vi "Main Editor UI.vi"() -> ()   [LabVIEW 2015, in "SystemLink editor node.lvclass"]
doc: "This is the main view for configuration the behavior of a module in the DCAF standard editor."
uses:
  SystemLink editor node.lvclass
  <vilib>/NI/Configuration Framework/Node/NodeRef.ctl
  <vilib>/NI/Configuration Framework/Node/NISE_CEF_Node.lvclass
  <vilib>/NI/AMC/Message Queue.ctl
  <vilib>/NI/AMC/Message.ctl
  <vilib>/NI/Tools/Keyed Array/KeyedArray.ctl
  <vilib>/NI/Configuration Framework/Node/UserEventRef.ctl
  <vilib>/NI/Configuration Framework/Controls/EventCluster.ctl
  <vilib>/NI/DCAF UI Toolkit/Controls/Configure.ctl
  <vilib>/NI/DCAF UI Toolkit/Controls/Add.ctl
  <vilib>/NI/DCAF UI Toolkit/Controls/Remove.ctl
  <vilib>/NI/Configuration Framework/Node/StopEvent.ctl
  <vilib>/NI/Configuration Framework/Node/RefreshUIEvent.ctl
  <vilib>/NI/Configuration Framework/Node/CacheState.ctl
  <vilib>/NI/Configuration Framework/Node/NodeChangeEvent.ctl
  module/configuration/Permissions Enum.ctl
  <vilib>/NI/DCAF/Tag Editor Core/Table API/Available Tag Menu/channel action event.ctl
  <vilib>/NI/DCAF/Tag Editor Core/Table API/Available Tag Menu/dialog output action.ctl
  <vilib>/NI/Tag Bus Module Framework/channel/TBM channel.lvclass
  <vilib>/NI/Tag Bus/tag/tag descriptor.lvclass
  <vilib>/NI/DCAF/Tag Editor Core/Table API/Table Manager/Call Back Ref Type Def.ctl
  <vilib>/NI/DCAF/Tag Editor Core/Configuration Editor/Classes/Engine Parent/Engine Parent Editor Node.lvclass
  <vilib>/NI/DCAF/Tag Editor Core/Configuration Editor/Classes/Module editor node/module editor node.lvclass
  <vilib>/NI/DCAF UI Toolkit/Controls/Import.ctl
  <vilib>/NI/DCAF UI Toolkit/Controls/Export.ctl
  module/configuration/Data Tag Type.ctl
  <vilib>/NI/DCAF/Tag Editor Core/Table API/Table Manager/references.ctl
  module/configuration/SystemLink configuration.lvclass
  module/configuration/SystemLink configuration.lvclass/SystemLink configuration.ctl
  <vilib>/Utility/miscctls.llb/LVPositionTypeDef.ctl
  module/configuration/Read Connection Configuration.vi
  <vilib>/NI/Configuration Framework/serializable configuration/NISE_CEF_serializable configuration.lvclass
  <vilib>/NI/DCAF/Tag Editor Core/Table API/Listbox/Multi Column Listbox.lvclass
  <vilib>/NI/Configuration Framework/NISE_CEF_TreeControl.lvlib
  <vilib>/NI/Tools/Keyed Array/Tools_KeyedArray.lvlib
  <vilib>/NI/AMC/AMC.lvlib
  <vilib>/NI/DCAF/Tag Editor Core/Table API/Table Manager.lvlib
  <vilib>/NI/DCAF/Tag Editor Core/Table API/Table Manager/Table Manager.lvclass
  <vilib>/NI/DCAF UI Toolkit/Controls/DCAF UI Elements.lvlib
panel:
  in  "Data Type":T1
  in  "user event out":refnum<user-event>
  in  "Permissions":T2
  in  "node change":T3
  in  "cache state":T4
  in  "refresh UI":T5
  in  "stop event":T6
  in  "Tab Control":T7(tab)=enum."Connection Configuration"
  in  "Remove Button":T8
  in  "Add Button":T9
  in  "Table":i32(listbox)
  in  "settings":T10
  in  "Configuration":T11={"Configuration ID"="", "HTTP"={"Verify Server?"=TRUE, "Server URL"="", "CA Certificate File"="", "User Info"={"Username"="", "Password"=""}, "API Key"=""}}
  in  "Connection Type":T12(ring)
  in  "Export":T13
  in  "Import":T14
  in  "user event":T15
  in  "main queue":T16
  in  "node ref":T17
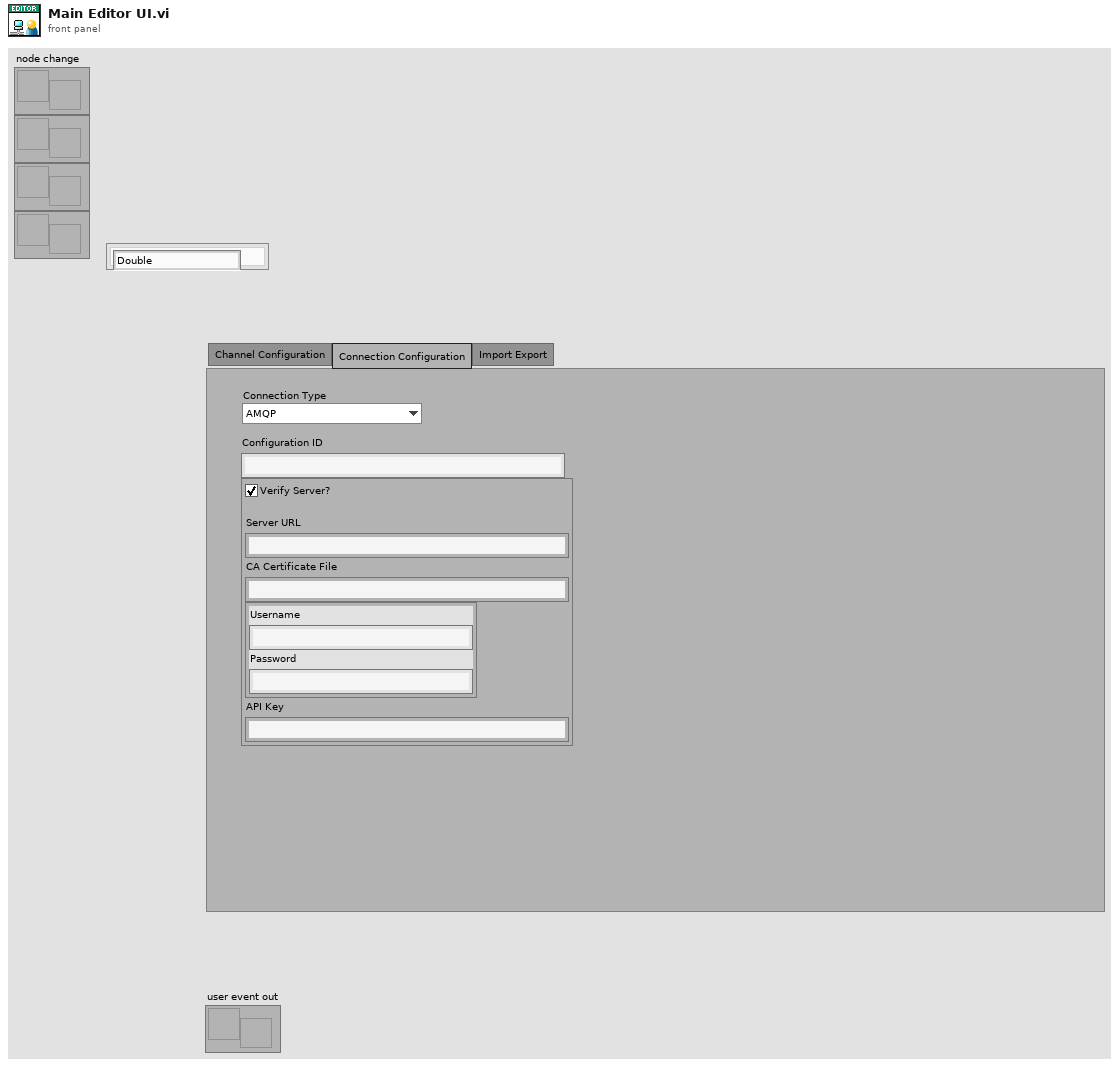
[diagram p1: front panel]
types:
  T1 = typedef "SystemLink configuration.lvclass/Data Tag Type.ctl" = enum16{"Double", "Single", "I32", "I16", "I8", "U64", "U32", "U16", "U8", "Boolean", "String", "Timestamp"}
  T2 = typedef "SystemLink configuration.lvclass/Permissions Enum.ctl" = enum16{"Read from SystemLink", "Write to SystemLink"}
  T3 = typedef "NISE_CEF_Node.lvclass/NodeChangeEvent.ctl" = refnum<user-event>
  T4 = typedef "NISE_CEF_Node.lvclass/CacheState.ctl" = refnum<user-event>
  T5 = typedef "NISE_CEF_Node.lvclass/RefreshUIEvent.ctl" = refnum<user-event>
  T6 = typedef "NISE_CEF_Node.lvclass/StopEvent.ctl" = refnum<user-event>
  T7 = enum32{"Channel Configuration", "Connection Configuration", "Import Export"}
  T8 = typedef "DCAF UI Elements.lvlib/Remove.ctl" = bool
  T9 = typedef "DCAF UI Elements.lvlib/Add.ctl" = bool
  T10 = typedef "DCAF UI Elements.lvlib/Configure.ctl" = bool
  T11 = cluster{"Configuration ID":string, "HTTP":cluster{"Verify Server?":bool, "Server URL":string, "CA Certificate File":string, "User Info":cluster{"Username":string, "Password":string}, "API Key":string}}
  T12 = enum16{"AMQP", "HTTP", "API Key (SystemLink Cloud)"}
  T13 = typedef "DCAF UI Elements.lvlib/Export.ctl" = bool
  T14 = typedef "DCAF UI Elements.lvlib/Import.ctl" = bool
  T15 = typedef "NISE_CEF_Node.lvclass/UserEventRef.ctl" = refnum<user-event>
  T16 = typedef "AMC.lvlib/Message Queue.ctl" = refnum<queue>
  T17 = typedef "NISE_CEF_Node.lvclass/NodeRef.ctl" = refnum<data-value>
  T18 = typedef "Table Manager.lvlib/Table Manager.lvclass/references.ctl" = cluster{"stop event":T6, "refresh UI":T5, "cache state":T4, "node change":T3, "user event out":refnum<user-event>, "main queue":T16, "user event":T15}
  T19 = typedef "LVPositionTypeDef.ctl" = cluster{"Left":i32, "Top":i32}
  T20 = typedef "Table Manager.lvlib/Table Manager.lvclass/object ref.ctl" = cluster{"engine":refnum<data-value>, "Node Ref":refnum<data-value>}
  T21 = typedef "Table Manager.lvlib/Column.lvclass/Column Descriptor.ctl" = cluster{"name":string, "caption":string, "Column Type":T22, "Params":string, "AutoSizeMode":i32, "FillWeight":sgl, "MinWidth":u32, "tooltip":string, "Enum Reference":refnum<vi>, "Channel suffix":string, "Read Only":bool, "Call Back VI":T23, "DT Dependency":i32, "name dependency":i32, "data type":T24, "Custom Column":refnum<class "Column.lvclass">}
  T22 = typedef "Table Manager.lvlib/Column.lvclass/Column Type.ctl" = enum16{"String", "Mapping", "Enum", "Custom"}
  T23 = typedef "Table Manager.lvlib/Table Manager.lvclass/Call Back Ref Type Def.ctl" = refnum<vi>
  T24 = typedef "tag bus.lvlib/tag descriptor.lvclass/Data Type.ctl" = enum16{"Double", "Single", "I64", "I32", "I16", "I8", "U64", "U32", "U16", "U8", "Boolean", "String", "Array of Double", "Array of Single", "Array of I64", "Array of I32", "Array of I16", "Array of I8", "Array of U64", "Array of U32", "Array of U16", "Array of U8", "Array of Boolean", "Array of String"}
  T25 = typedef "SystemLink configuration.lvclass/Connection Configuration.ctl" = cluster{"Connection Type":T26, "AMQP":cluster{"Configuration ID":string}, "HTTP":cluster{"Verify Server?":bool, "Server URL":string, "CA Certificate File":string, "User Info":cluster{"Username":string, "Password":string}, "API Key":string}}
  T26 = typedef "SystemLink configuration.lvclass/Connection Type.ctl" = enum16{"AMQP", "HTTP", "API Key (SystemLink Cloud)"}
  T27 = cluster{"Verify Server?":bool, "Server URL":string, "CA Certificate File":string, "User Info":cluster{"Username":string, "Password":string}, "API Key":string}
  T28 = typedef "Table Manager.lvlib/Table Manager.lvclass/Table Events.ctl" = cluster{"Menu Selection":refnum<user-event>}
  T29 = enum8{"Enabled", "Disabled", "Disabled and Grayed Out"}
  T30 = cluster{"AMQP Specific":refnum<vi>, "HTTP Generic":refnum<vi>, "HTTP Specific":refnum<vi>, "API Key Specific":refnum<vi>}
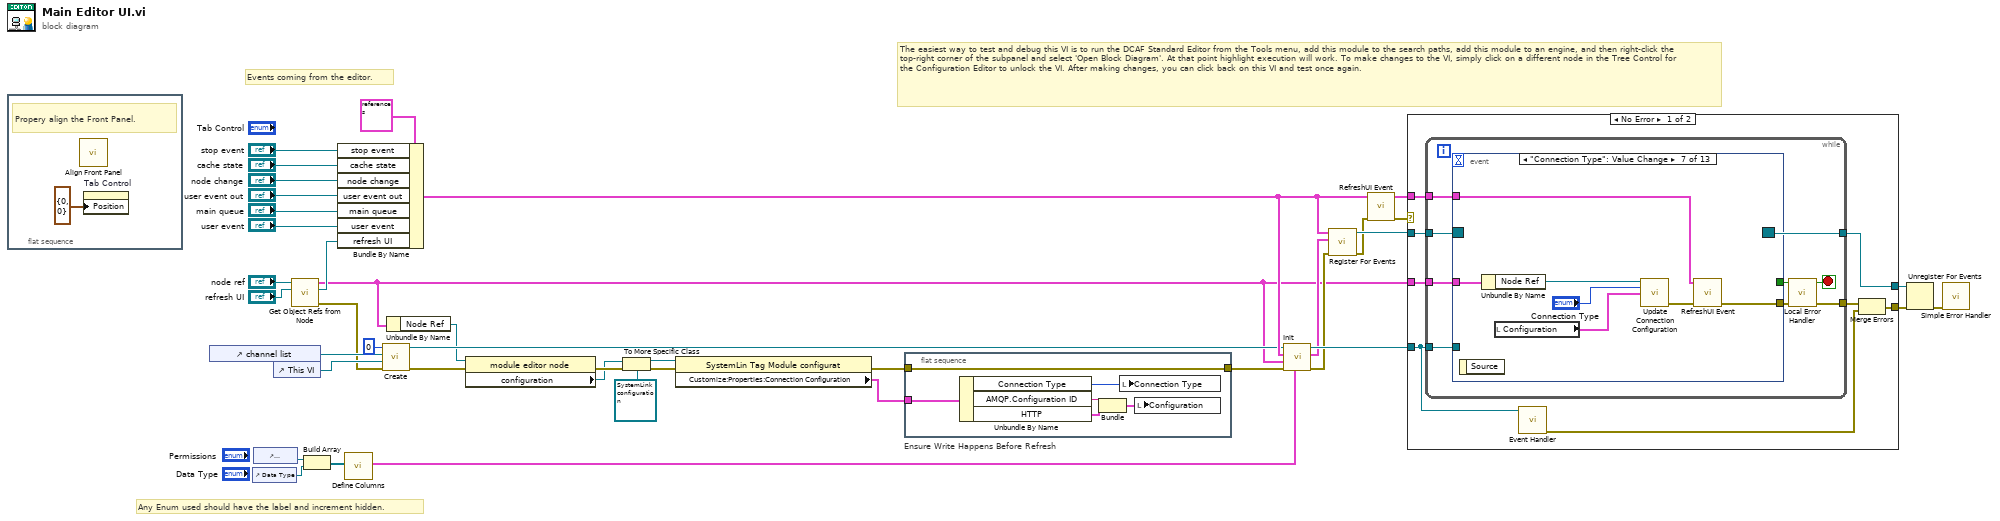
[diagram p0: block diagram]
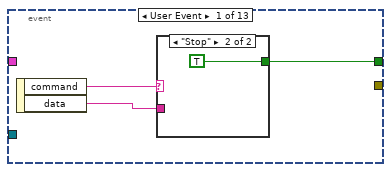
[diagram p2: hidden frame]
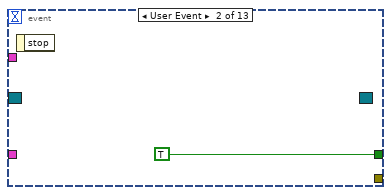
[diagram p4: hidden frame]
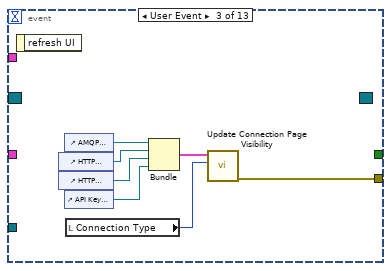
[diagram p5: hidden frame]
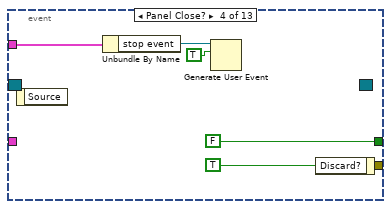
[diagram p6: hidden frame]
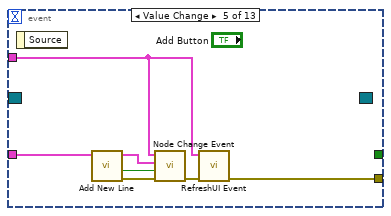
[diagram p7: hidden frame]
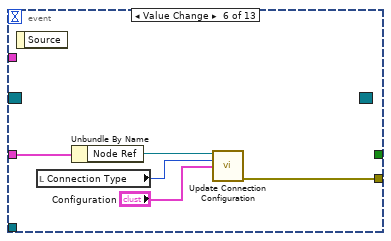
[diagram p8: hidden frame]
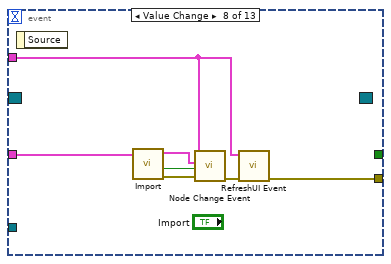
[diagram p9: hidden frame]
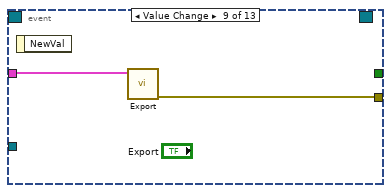
[diagram p10: hidden frame]
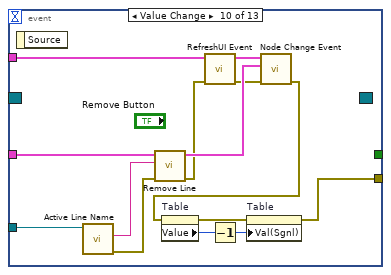
[diagram p11: hidden frame]
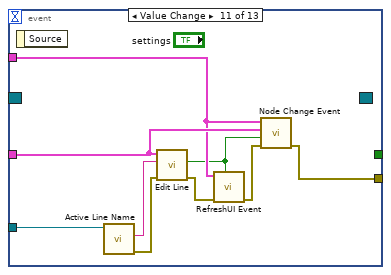
[diagram p12: hidden frame]
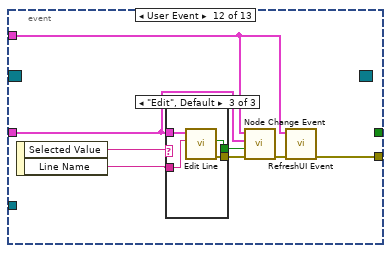
[diagram p13: hidden frame]
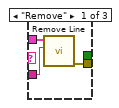
[diagram p14: hidden frame]
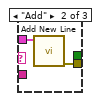
[diagram p15: hidden frame]
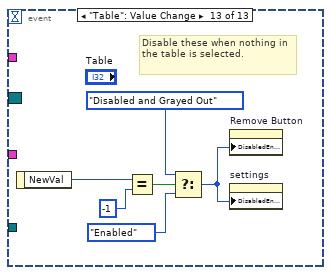
[diagram p16: hidden frame]
diagram:
  # "The easiest way to test and debug this VI is to run the DCAF Standard Editor from the Tools menu, add this module to the search paths, add this module to an engine, and then right-click the top-right corner of the subpanel and select 'Open Block Diagram'. At that point highlight execution will work. To make changes to the VI, simply click on a different node in the Tree Control for the Configuration Editor to unlock the VI. After making changes, you can click back on this VI and test once again."
  # "Any Enum used should have the label and increment hidden."
  # "Events coming from the editor."
  n1 = flat-sequence {
    frame #0 {
      # "Propery align the Front Panel."
      n2 = call <vilib>:"Align Front Panel.vi"() -> ()  [unwired: 10 in, 2 out]
      n3 = property on="Tab Control" class="TabCtl (strict)"("Position"=T19 {"Left"=0, "Top"=0}) -> ()  [unwired: 2 in, 2 out]
    }
  }
  n4 = control-ref of="channel list"() -> (w19:refnum<vi>)
  n5 = control-ref of="Data Type"() -> (w11:refnum<vi>)
  n6 = control-ref of="Permissions"() -> (w27:refnum<vi>)
  n7 = control-ref of="This VI"() -> (w17:refnum<vi>)
  n8 = call "Get Object Refs from Node.vi"("Refresh UI"="refresh UI", "Data Value Reference in"="node ref") -> ("error out"=w14:errorcluster, "Refresh UI out"=w12:T5, "References"=w9:T20)  [unwired: 7 in]
  n9 = Build Array(w27, w11) -> (w26:refnum<vi>[])
  n10 = Bundle By Name(cluster=T18 {"stop event"=refnum, "refresh UI"=refnum, "cache state"=refnum, "node change"=refnum, "user event out"=refnum, "main queue"=refnum, "user event"=refnum} ("References"), "stop event"="stop event", "cache state"="cache state", "node change"="node change", "user event out"="user event out", "main queue"="main queue", "user event"="user event", "refresh UI"=w12) -> (w28:T18)
  n11 = call "Define Columns.vi"("Enum Array"=w26) -> ("Column Definition"=w30:T21[])  [unwired: 10 in]
  n12 = call <vilib>:"Create.vi"("error in (no error)"=w14, "Top VI"=w17, "Listbox"=w19, "Index"=0) -> ("error out"=w15:errorcluster, "reference out"=w16:refnum<class "Multi Column Listbox.lvclass">)  [unwired: 6 in]
  n13 = Unbundle By Name(w9) -> ("Node Ref"=w8:refnum<data-value>)
  n14 = property class="module editor node"(reference=w8, error in=w15) -> (error out=w10:errorcluster, "configuration"=w6:refnum<class "NISE_CEF_serializable configuration.lvclass">)  [unwired: 1 out]
  n15 = To More Specific Class(target class=refnum<class "SystemLink configuration.lvclass"> refnum ("SystemLin Tag Module configuration"), reference=w6, error in=w10) -> (specific class reference=w4:refnum<class "SystemLink configuration.lvclass">, error out=w7:errorcluster)
  n16 = property class="SystemLin Tag Module configurat"(reference=w4, error in=w7) -> (error out=w2:errorcluster, "Customize:Properties:Connection Configuration"=w3:T25)  [unwired: 1 out]
  n17 = flat-sequence "Ensure Write Happens Before Refresh" {
    tunnel: w3 -> [w48]
    tunnel: w2 -> [w46]
    tunnel: [w46] -> w1
    frame #0 {
      n18 = Unbundle By Name(w48) -> ("Connection Type"=w47:T26, "AMQP.Configuration ID"=w44:string, "HTTP"=w43:T27)
      n19 = Bundle("Configuration ID"=w44, "HTTP"=w43) -> (w45:T11)  [unwired: 1 in]
      n20 = local write "Connection Type"(w47) -> ()
      n21 = local write "Configuration"(w45) -> ()
    }
  }
  n22 = call-dynamic "Init.vi"("Column Descriptors"=w30, "error in (no error)"=w1, "Node object refs"=w9, "Event References"=w28, "Multi Column Listbox in"=w16) -> ("error out"=w21:errorcluster, "Table Events"=w20:T28, "Multi Column Listbox out"=w25:refnum<class "Multi Column Listbox.lvclass">)  [unwired: 4 in]
  n23 = call "Register For Events.vi"("error in"=w21, "Table Events"=w20, "References"=w28) -> ("error out"=w23:errorcluster, "Event Registration Refnum"=w31:refnum<event-registration>)  [unwired: 7 in]
  n24 = call "RefreshUI Event.vi"("error in (no error)"=w23, "References in"=w28) -> ("error out"=w22:errorcluster, "References out"=w29:T18)  [unwired: 8 in]
  n25 = case shown="No Error" w22 {
    selector: w22 -> [_ w156]
    tunnel: w31 -> [w56 w155]
    tunnel: [w55 w155] -> w41
    tunnel: [w49 w156] -> w40
    tunnel: w29 -> [w54 _]
    tunnel: w9 -> [w53 _]
    tunnel: w25 -> [w52 _]
    frame No Error {
      n26 = while {
        tunnel: w56 -> [w65]
        tunnel: [w64] -> w55
        tunnel: [w61] -> w50
        tunnel: w54 -> [w59]
        tunnel: w53 -> [w58]
        tunnel: w52 -> [w57]
        stop <- w63 stop-if-true
        n27 = event shown="[6] \"Connection Type\": Value Change" {
          selector: w65 -> [_ _ _ _ _ _ _ _ _ _ _ _ _]
          dyn-events: [_ _ _ _ _ _ _ _ _ _ _ _ _] -> w64
          timeout: _ -> [_ _ _ _ _ _ _ _ _ _ _ _ _]
          tunnel: [w68 TRUE _ FALSE _ _ _ _ _ _ _ _ _] -> w62
          tunnel: [_ _ w71 _ w83 w91 w96 w106 w109 w111 w131 w137 _] -> w60
          tunnel: w59 -> [_ _ _ w79 w87 _ w95 w103 _ w122 w126 w133 _]
          tunnel: w58 -> [_ _ _ _ w88 w93 w99 w105 w108 w121 w129 w134 _]
          tunnel: w57 -> [_ _ _ _ _ _ _ _ _ w117 w130 _ _]
          event User Event {
            n28 = event-data() -> ("command"=w67:string, "data"=w66:string)  [unwired: 1 in]
            n29 = case shown="\"Stop\"" w67 {
              tunnel: [_ TRUE] -> w68
              tunnel: w66 -> [_ _]
              frame Default {
              }
              frame "Stop" {
              }
            }
          }
          event User Event {
            n30 = event-data() -> ()  [unwired: 1 in, 1 out]
          }
          event User Event {
            n31 = event-data() -> ()  [unwired: 1 in, 1 out]
            n32 = control-ref of="HTTP Generic"() -> (w76:refnum<vi>)
            n33 = control-ref of="HTTP Specific"() -> (w75:refnum<vi>)
            n34 = control-ref of="AMQP Specific"() -> (w77:refnum<vi>)
            n35 = control-ref of="API Key Specific"() -> (w74:refnum<vi>)
            n36 = local read "Connection Type"() -> (w72:T12)
            n37 = Bundle("AMQP Specific"=w77, "HTTP Generic"=w76, "HTTP Specific"=w75, "API Key Specific"=w74) -> (w73:T30)  [unwired: 1 in]
            n38 = call "Update Connection Page Visibility.vi"("Connection Type"=w72, "Config References"=w73) -> ("error out"=w71:errorcluster)  [unwired: 9 in]
          }
          event Panel Close? {
            n39 = event-data() -> ()  [unwired: 1 in, 1 out]
            n40 = Unbundle By Name(w79) -> ("stop event"=w78:T6)
            n41 = Generate User Event(user event=w78, event data cluster=TRUE ("event data")) -> ()  [unwired: 2 in, 2 out]
            n42 = event-data("Discard?"=TRUE) -> ()  [unwired: 1 in, 1 out]
          }
          event Value Change {
            n43 = event-data() -> ()  [unwired: 1 in, 1 out]
            n44 = call "Add New Line.vi"("objects"=w88) -> ("error out"=w86:errorcluster, "success"=w84:bool)  [unwired: 8 in, 1 out]
            n45 = call "Node Change Event.vi"("error in (no error)"=w86, "Send (T)"=w84, "objects"=w88, "References in"=w87) -> ("error out"=w85:errorcluster)  [unwired: 7 in]
            n46 = call "RefreshUI Event.vi"("error in (no error)"=w85, "References in"=w87) -> ("error out"=w83:errorcluster)  [unwired: 8 in, 1 out]
          }
          event "Configuration.HTTP", "Configuration.Configuration ID": Value Change {
            n47 = event-data() -> ()  [unwired: 1 in, 1 out]
            n48 = local read "Connection Type"() -> (w90:T12)
            n49 = Unbundle By Name(w93) -> ("Node Ref"=w92:refnum<data-value>)
            n50 = call "Update Connection Configuration.vi"("Data Value Reference in"=w92, "Connection Type"=w90, "Configuration"="Configuration") -> ("error out"=w91:errorcluster)  [unwired: 12 in]
          }
          event "Connection Type": Value Change {
            n51 = event-data() -> ()  [unwired: 1 in, 1 out]
            n52 = Unbundle By Name(w99) -> ("Node Ref"=w100:refnum<data-value>)
            n53 = local read "Configuration"() -> (w94:T11)
            n54 = call "Update Connection Configuration.vi"("Data Value Reference in"=w100, "Connection Type"="Connection Type", "Configuration"=w94) -> ("error out"=w97:errorcluster)  [unwired: 12 in]
            n55 = call "RefreshUI Event.vi"("error in (no error)"=w97, "References in"=w95) -> ("error out"=w96:errorcluster)  [unwired: 8 in, 1 out]
          }
          event Value Change {
            n56 = event-data() -> ()  [unwired: 1 in, 1 out]
            n57 = call "Import.vi"("Objects in"=w105) -> ("error out"=w102:errorcluster, "Update"=w101:bool, "Objects out"=w104:T20)  [unwired: 8 in]
            n58 = call "Node Change Event.vi"("error in (no error)"=w102, "Send (T)"=w101, "objects"=w104, "References in"=w103) -> ("error out"=w107:errorcluster)  [unwired: 7 in]
            n59 = call "RefreshUI Event.vi"("error in (no error)"=w107, "References in"=w103) -> ("error out"=w106:errorcluster)  [unwired: 8 in, 1 out]
          }
          event Value Change {
            n60 = event-data() -> ()  [unwired: 1 in, 1 out]
            n61 = call "Export.vi"("Objects"=w108) -> ("error out"=w109:errorcluster)  [unwired: 10 in]
          }
          event Value Change {
            n62 = event-data() -> ()  [unwired: 1 in, 1 out]
            n63 = call-dynamic "Active Line Name.vi"("Multi Column Listbox in"=w117) -> ("error out"=w115:errorcluster, "Active Line Name"=w116:string)  [unwired: 8 in, 1 out]
            n64 = call "Remove Line.vi"("error in"=w115, "Active Line Name"=w116, "Objects"=w121) -> ("error out"=w118:errorcluster)  [unwired: 8 in]
            n65 = call "RefreshUI Event.vi"("error in (no error)"=w118, "References in"=w122) -> ("error out"=w120:errorcluster, "References out"=w119:T18)  [unwired: 8 in]
            n66 = call "Node Change Event.vi"("error in (no error)"=w120, "objects"=w121, "References in"=w119) -> ("error out"=w112:errorcluster)  [unwired: 8 in]
            n67 = property on="Table" class="MCListbox (strict)"(error in=w112) -> (error out=w110:errorcluster, "Value"=w113:i32)  [unwired: 1 in, 1 out]
            n68 = Decrement(x=w113) -> (x-1=w114:i32)
            n69 = property on="Table" class="MCListbox (strict)"(error in=w110, "Val(Sgnl)"=w114) -> (error out=w111:errorcluster)  [unwired: 1 in, 1 out]
          }
          event Value Change {
            n70 = event-data() -> ()  [unwired: 1 in, 1 out]
            n71 = call-dynamic "Active Line Name.vi"("Multi Column Listbox in"=w130) -> ("error out"=w127:errorcluster, "Active Line Name"=w128:string)  [unwired: 8 in, 1 out]
            n72 = call "Edit Line.vi"("error in"=w127, "Line Name"=w128, "References"=w129) -> ("error out"=w124:errorcluster, "change?"=w125:bool)  [unwired: 7 in]
            n73 = call "RefreshUI Event.vi"("Refresh (T)"=w125, "error in (no error)"=w124, "References in"=w126) -> ("error out"=w123:errorcluster)  [unwired: 7 in, 1 out]
            n74 = call "Node Change Event.vi"("error in (no error)"=w123, "Send (T)"=w125, "objects"=w129, "References in"=w126) -> ("error out"=w131:errorcluster)  [unwired: 7 in]
          }
          event User Event {
            n75 = event-data() -> ("Selected Value"=w139:string, "Line Name"=w136:string)  [unwired: 1 in]
            n76 = case shown="\"Edit\", Default" w139 {
              tunnel: w136 -> [w142 _ w148]
              tunnel: w134 -> [w141 w144 w147]
              tunnel: [w140 w143 w146] -> w135
              tunnel: [_ _ w145] -> w132
              frame "Remove" {
                n77 = call "Remove Line.vi"("Active Line Name"=w142, "Objects"=w141) -> ("error out"=w140:errorcluster)  [unwired: 9 in]
              }
              frame "Add" {
                n78 = call "Add New Line.vi"("objects"=w144) -> ("error out"=w143:errorcluster)  [unwired: 8 in, 2 out]
              }
              frame "Edit", Default {
                n79 = call "Edit Line.vi"("Line Name"=w148, "References"=w147) -> ("error out"=w146:errorcluster, "change?"=w145:bool)  [unwired: 8 in]
              }
            }
            n80 = call "Node Change Event.vi"("error in (no error)"=w135, "Send (T)"=w132, "objects"=w134, "References in"=w133) -> ("error out"=w138:errorcluster)  [unwired: 7 in]
            n81 = call "RefreshUI Event.vi"("error in (no error)"=w138, "References in"=w133) -> ("error out"=w137:errorcluster)  [unwired: 8 in, 1 out]
          }
          event "Table": Value Change {
            # "Disable these when nothing in the table is selected."
            n82 = event-data() -> ("NewVal"=w154:i32)  [unwired: 1 in]
            n83 = Equal?(x=w154, y=-1) -> (x = y?=w152:bool)
            n84 = Select(t=T29."Disabled and Grayed Out" ("Disabled"), s=w152, f=T29."Enabled") -> (s? t:f=w150:T29)
            n85 = property on="Remove Button" class="Bool"("DisabledEnum"=w150) -> ()  [unwired: 2 in, 2 out]
            n86 = property on="settings" class="Bool"("DisabledEnum"=w150) -> ()  [unwired: 2 in, 2 out]
          }
        }
        n87 = call "Local Error Handler.vi"("error in"=w60, "Stop in"=w62) -> ("error out"=w61:errorcluster, "Stop out"=w63:bool)  [unwired: 8 in]
      }
      n88 = call-dynamic "Event Handler.vi"("Listbox in"=w52) -> ("error out"=w51:errorcluster)  [unwired: 9 in, 1 out]
      n89 = Merge Errors(w50, w51) -> (w49:errorcluster)
    }
    frame Error {
    }
  }
  n90 = Unregister For Events(event registration refnum=w41, error in=w40) -> (error out=w39:errorcluster)
  n91 = call <vilib>:"Simple Error Handler.vi"("error in (no error)"=w39) -> ()  [unwired: 4 in, 5 out]
